vi "Write Include or Exclude.vi"(10 "Include or Exclude":enum16{"Include", "Exclude"}(ring), 11 "Base Filter in":refnum<class "Base Filter.lvclass">) -> (3 "Base Filter out":refnum<class "Base Filter.lvclass">)   [LabVIEW 2016, in "Assert API Components.lvlib" / "Base Filter.lvclass"]
uses:
  Base Filter.lvclass
  Base Filter.lvclass/Base Filter.ctl
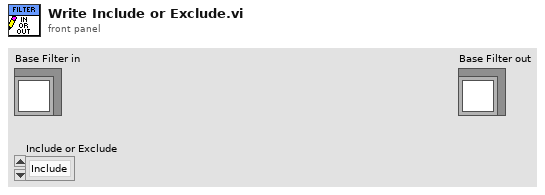
[diagram p1: front panel]
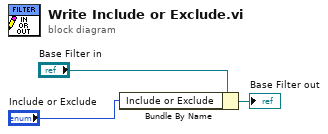
[diagram p0: block diagram]
diagram:
  n1 = Bundle By Name(cluster="Base Filter in", "Include or Exclude"="Include or Exclude") -> (→"Base Filter out":refnum<class "Base Filter.lvclass">)
